vi "例程18-绘制单位球面.vi"() -> ()   [LabVIEW 2016]
uses:
  <vilib>/Platform/NI_3dgraph.lvlib
panel:
  in  "3D Parametric Surface":refnum<k7>(container) caption="三维参数曲面"
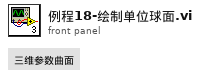
[diagram p1: front panel]
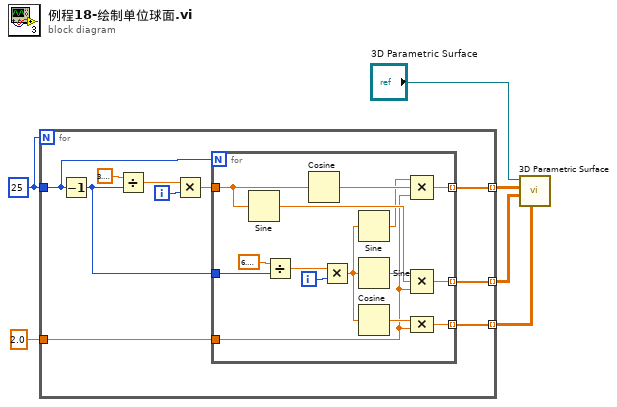
[diagram p0: block diagram]
diagram:
  w6 = 25
  n1 = for {
    N: w6 -> [_]
    tunnel: w6 -> [w11]
    tunnel: [w13] -> w3 mode=indexing
    tunnel: [w12] -> w4 mode=indexing
    tunnel: [w8] -> w2 mode=indexing
    tunnel: 2.0 ("值") -> [w7]
    i -> [w10]
    n2 = Decrement(x=w11) -> (x-1=w9:i32)
    n3 = Divide(x=3.141592653589793, y=w9) -> (x/y=w16:dbl)
    n4 = Multiply(x=w16, y=w10) -> (x*y=w14:dbl)
    n5 = for {
      N: w11 -> [_]
      tunnel: w9 -> [w30]
      tunnel: w14 -> [w27]
      tunnel: [w22] -> w12 mode=indexing
      tunnel: [w20] -> w13 mode=indexing
      tunnel: [w18] -> w8 mode=indexing
      tunnel: w7 -> [w17]
      i -> [w29]
      n6 = Sine(x=w27) -> (sin(x)=w26:dbl)
      n7 = Divide(x=6.283185307179586, y=w30) -> (x/y=w28:dbl)
      n8 = Cosine(x=w27) -> (cos(x)=w24:dbl)
      n9 = Multiply(x=w28, y=w29) -> (x*y=w21:dbl)
      n10 = Sine(x=w21) -> (sin(x)=w23:dbl)
      n11 = Sine(x=w21) -> (sin(x)=w25:dbl)
      n12 = Cosine(x=w21) -> (cos(x)=w19:dbl)
      n13 = Compound Arithmetic op=MULTIPLY(w23, w24, w17) -> (w22:dbl)
      n14 = Compound Arithmetic op=MULTIPLY(w25, w26, w17) -> (w20:dbl)
      n15 = Compound Arithmetic op=MULTIPLY(w19, w17) -> (w18:dbl)
    }
  }
  n16 = call <vilib>:"3D Parametric Surface.vi"("z matrix"=w2, "y matrix"=w3, "x matrix"=w4, "3D graph"="3D Parametric Surface") -> ()  [unwired: 6 in, 2 out]
